vi "UDP 읽기02.vi"() -> ()   [LabVIEW 2014]
panel:
  in  "정지":bool
  out "데이터 출력":string
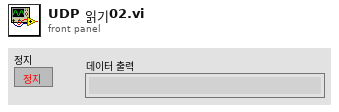
[diagram p1: front panel]
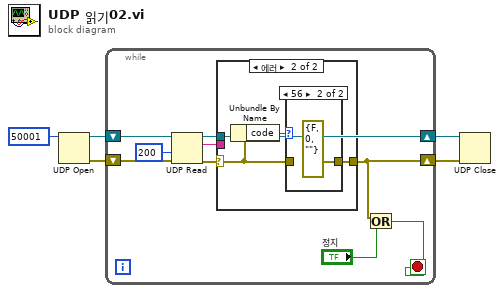
[diagram p0: block diagram]
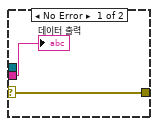
[diagram p2: hidden frame]
diagram:
  n1 = UDP Open(11:u16 50001 ("포트")) -> (port=w5:refnum<k16>, 0:w3:errorcluster)  [unwired: 4 in, 1 out]
  n2 = while {
    shift-right: [w6] -> w4
    shift-left: w5 -> [w14]
    shift-right: [w7] -> w2
    shift-left: w3 -> [w13]
    stop <- w11 stop-if-true
    n3 = UDP Read(connection ID=w14, timeout ms (25000)=200 ("타임아웃 ms (25000)"), 8:w13) -> (data out=w12:string, error out=w8:errorcluster, 3:w6:refnum<k16>)  [unwired: 1 in, 2 out]
    n4 = case shown="에러" w8 {
      selector: w8 -> [w15 w17]
      tunnel: w12 -> [w16 _]
      tunnel: [w15 w18] -> w7
      tunnel: w6 -> [_ _]
      frame No Error {
        "데이터 출력" <- w16
      }
      frame Error {
        n5 = Unbundle By Name(w17) -> ("code"=w19:i32)
        n6 = case shown="56" w19 {
          tunnel: [w20 errorcluster {"status"=FALSE, "code"=0, "source"=""} ("에러 상수")] -> w18
          tunnel: w17 -> [w20 _]
          frame Default {
          }
          frame 56 {
          }
        }
      }
    }
    n7 = Or(x=w7, y="정지") -> (x .or. y?=w11:bool)
  }
  n8 = UDP Close(connection ID=w4, 8:w2) -> ()  [unwired: 2 out]
